vi "number1_sub1-data acquisition.vi"() -> (1 "Waveform Graph":waveform(dbl)(graph))   [LabVIEW 2014]
uses:
  number1_global.vi
  <vilib>/measure/NI_MABase.lvlib
panel:
  out "#s":dbl
  in  "OK Button":bool
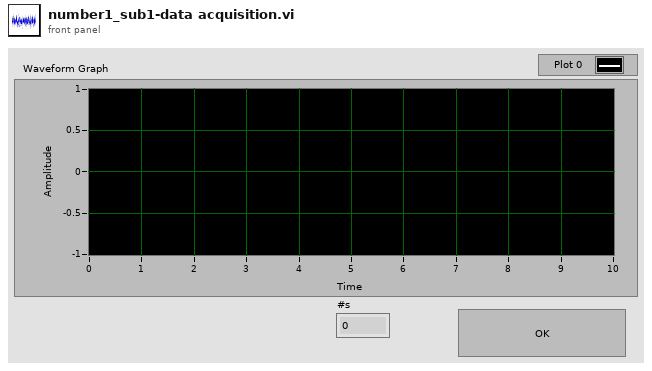
[diagram p1: front panel]
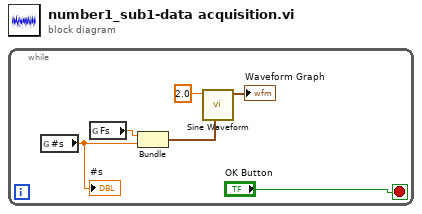
[diagram p0: block diagram]
diagram:
  n1 = while {
    stop <- "OK Button" stop-if-true
    n2 = global read "number1_global.vi" "#s"() -> (w2:dbl)
    "#s" <- w2
    n3 = global read "number1_global.vi" "Fs"() -> (w3:dbl)
    n4 = Bundle("Fs"=w3, "#s"=w2) -> (w5:cluster{"Fs":dbl, "#s":dbl})  [unwired: 1 in]
    n5 = call <vilib>:"Sine Waveform.vi"("sampling info"=w5, "frequency"=2.0) -> ("signal out"=→"Waveform Graph":waveform(dbl))  [unwired: 8 in, 1 out]
  }
